vi "WebServices path--constant.vi"() -> (3 "WebServices path":path)   [LabVIEW 2020, in "WSsupport.lvlib"]
uses:
  WSsupport.lvlib
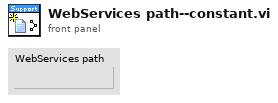
[diagram p1: front panel]
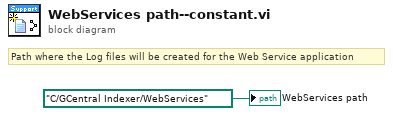
[diagram p0: block diagram]
diagram:
  # "Path where the Log files will be created for the Web Service application"
  "WebServices path" <- path "C:/GCentral Indexer/WebServices" ("base path")
